vi "sv_Fractional Octave Filtering (1 Ch).vi"(0 "scaled signal [EU]":waveform(dbl), 1 "reset filter (F)":bool, 5 "1/n octave settings":T3, 7 "midband frequency setting":T1, 11 "error in (no error)":errorcluster) -> (4 "filtered signal [EU]":waveform(dbl), 6 "settled?":bool, 8 "actual midband frequency [Hz]":dbl, 15 "error out":errorcluster)   [LabVIEW 2017, in "SoundVib_Octave_2014 standard.lvlib"]
doc: "This VI designs a single octave filter based on the specified midband frequency and bandwidth and applies the filter to input time domain signal.\n\nThe fractional-octave filter is designed in accordance with one of the following standards:\n ANSI S1.11-2014;\n IEC 61260-1:2014.\nFor both standards, the sampling frequency must be at least 3 times the highest midband frequency for octave analysis and at least 2.5 times the highest midband frequency for 1/3, 1/6, 1/12, or 1/24 octave analysis. Available bandwidths are 1/1, 1/3, 1/6, 1/12, and 1/24 octave.\n\nTo ensure a continuous filtering operation, call this VI the first time with reset filter set to TRUE and then call it with reset filter set to FALSE.\n\nTo design a standard octave filter, set coerce to nearest standard midband frequency to TRUE."
uses:
  <vilib>/addons/Sound and Vibration/svt_Octave/SoundVib_Octave_2014 standard.lvlib
  <vilib>/addons/_NISVFA/_Shared subVIs/Controls/svc_Octave Standard.ctl
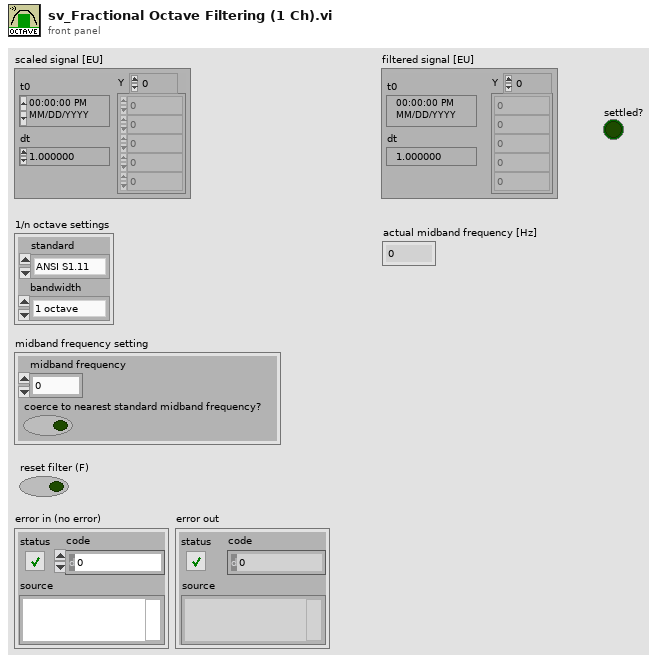
[diagram p1: front panel]
types:
  T1 = cluster{"midband frequency":dbl, "coerce to nearest standard midband frequency?":bool}
  T2 = typedef "svc_Octave Standard.ctl" = enum16{"ANSI S1.11", "IEC 61260"}
  T3 = cluster{"standard":T2, "bandwidth":enum16{"1 octave", "1/3 octave", "1/6 octave", "1/12 octave", "1/24 octave"}}
  T4 = enum16{"1 octave", "1/3 octave", "1/6 octave", "1/12 octave", "1/24 octave"}
  T5 = typedef "svc_Octave Filter Bank Parameters.ctl" = cluster{"octave filter coefficients":cluster{"filter structure":enum32{"IIR 2nd Order", "IIR 4th Order"}, "Reverse Coefficients":dbl[], "Forward Coefficients":dbl[]}[], "lowpass filter coefficients":cluster{"filter structure":enum32{"IIR 2nd Order", "IIR 4th Order"}, "Reverse Coefficients":dbl[], "Forward Coefficients":dbl[]}, "number of samples to settle":u64, "number of decimation steps required":i32[], "octave filter bandwidth":dbl[]}
  T6 = typedef "svc_Octave Filter State.ctl" = cluster{"octave filter":cluster{"Octave filter":dbl[]}[], "lowpass filter":dbl[][], "exponential averaging":cluster{"exponential averaging":dbl, "peak detector":dbl}[], "linear averaging":cluster{"squared sum":dbl, "size":dbl}[], "result":dbl[], "number of samples since init":u64, "decimation":dbl[]}
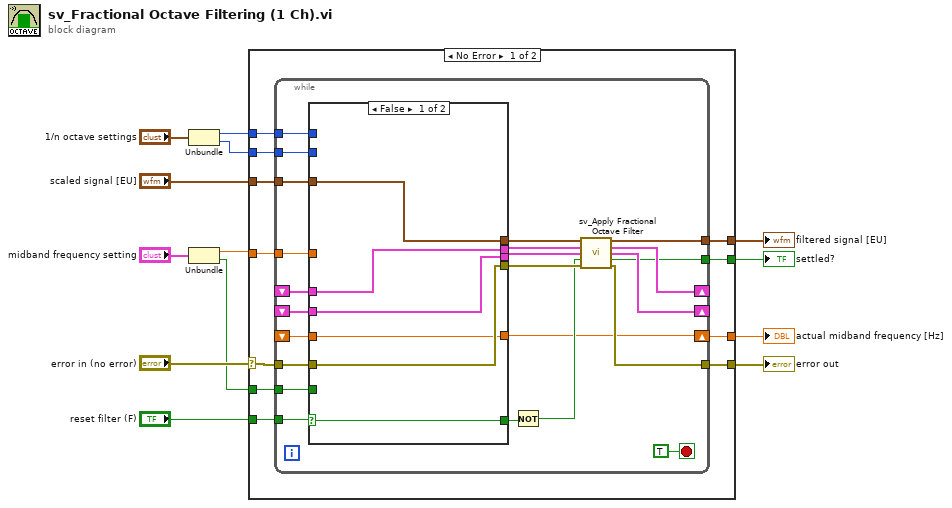
[diagram p0: block diagram]
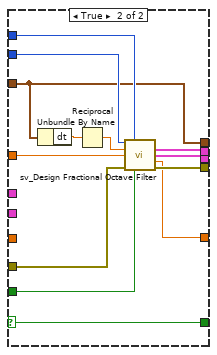
[diagram p2: hidden frame]
diagram:
  n1 = Unbundle("1/n octave settings") -> ("standard"=w6:T2, "bandwidth"=w5:T4)
  n2 = Unbundle("midband frequency setting") -> ("midband frequency"=w2:dbl, "coerce to nearest standard midband frequency?"=w3:bool)
  n3 = case shown="No Error" "error in (no error)" {
    selector: "error in (no error)" -> [w18 w67]
    tunnel: w2 -> [w24 _]
    tunnel: w3 -> [w23 _]
    tunnel: w5 -> [w22 _]
    tunnel: w6 -> [w21 _]
    tunnel: "scaled signal [EU]" -> [w20 _]
    tunnel: [w16 w67] -> w12
    tunnel: "reset filter (F)" -> [w19 _]
    tunnel: [w17 _] -> w9
    tunnel: [w15 _] -> w8
    tunnel: [w14 _] -> w1
    frame No Error {
      n4 = while {
        tunnel: w24 -> [w47]
        tunnel: w23 -> [w46]
        tunnel: w22 -> [w45]
        tunnel: w21 -> [w44]
        tunnel: w19 -> [w40]
        tunnel: w18 -> [w42]
        tunnel: w20 -> [w43]
        shift-right: [w29] -> _
        shift-left: _ -> [w38]
        shift-right: [w30] -> _
        shift-left: _ -> [w37]
        tunnel: [w31] -> w17
        tunnel: [w28] -> w16
        tunnel: [w27] -> w15
        shift-right: [w26] -> w14
        shift-left: _ -> [w25]
        stop <- TRUE stop-if-true
        n5 = case shown="False" w40 {
          selector: w40 -> [w52 w59]
          tunnel: w47 -> [_ w66]
          tunnel: w46 -> [_ w65]
          tunnel: w45 -> [_ w64]
          tunnel: w44 -> [_ w63]
          tunnel: w43 -> [w53 w60]
          tunnel: w42 -> [w51 w62]
          tunnel: [w51 w61] -> w36
          tunnel: [w53 w60] -> w35
          tunnel: [w52 w59] -> w39
          tunnel: w38 -> [w49 _]
          tunnel: w37 -> [w50 _]
          tunnel: [w50 w57] -> w33
          tunnel: [w49 w56] -> w34
          tunnel: [w48 w54] -> w26
          tunnel: w25 -> [w48 _]
          frame False {
          }
          frame True {
            n6 = Unbundle By Name(w60) -> ("dt"=w58:dbl)
            n7 = Reciprocal(x=w58) -> (1/x=w55:dbl)
            n8 = call <vilib>:"sv_Design Fractional Octave Filter.vi"("bandwidth"=w64, "standard"=w63, "sampling frequency [Hz]"=w55, "midband frequency [Hz]"=w66, "error in (no error)"=w62, "coerce to nearest standard midband frequency?"=w65) -> ("filter bank parameters"=w56:T5, "initial filter state"=w57:T6, "actual midband frequency [Hz]"=w54:dbl, "error out"=w61:errorcluster)  [unwired: 5 in, 1 out]
          }
        }
        n9 = Not(x=w39) -> (.not. x?=w32:bool)
        n10 = call <vilib>:"sv_Apply Fractional Octave Filter.vi"("scaled signal [EU]"=w35, "filter bank parameters"=w34, "internal filter state IN"=w33, "filter init/cont (init:F)"=w32, "error in (no error)"=w36) -> ("filtered data"=w31:waveform(dbl), "dup filter bank parameters"=w29:T5, "internal filter state OUT"=w30:T6, "settled?"=w27:bool, "error out"=w28:errorcluster)  [unwired: 6 in]
      }
    }
    frame Error {
    }
  }
  "error out" <- w12
  "filtered signal [EU]" <- w9
  "settled?" <- w8
  "actual midband frequency [Hz]" <- w1
